vi "Process Menu Selection.vi"(8 "error in (no error)":errorcluster, 10 "Argument":string, 11 "Menu Ref":refnum<k9>) -> (0 "error out":errorcluster, 3 "State(s) to Enqueue":string)   [LabVIEW 2023, in "VI Properties Editor.lvlib"]
doc: "Processes a menu selection that occurred within the main window."
uses:
  VI Properties Editor.lvlib
  <vilib>/Utility/error.llb/Error Cluster From Error Code.vi
  <vilib>/ErrorRing/Error Ring.xnode
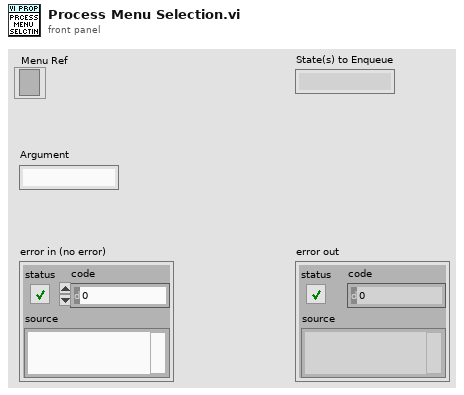
[diagram p1: front panel]
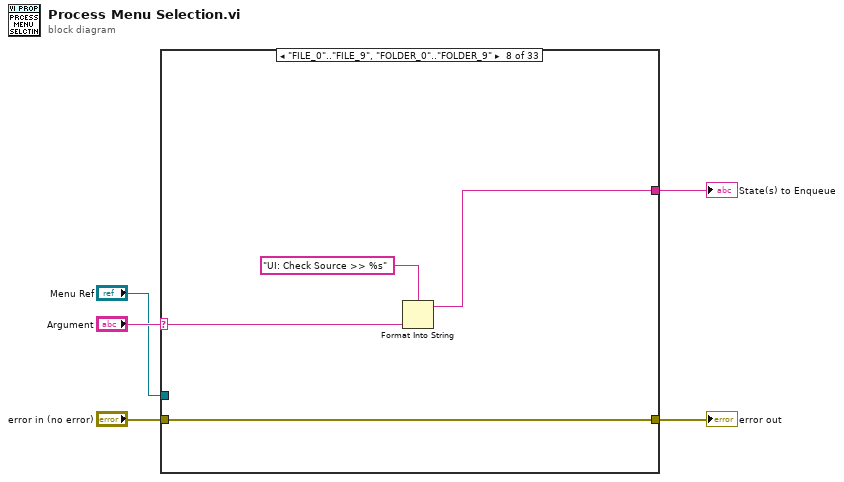
[diagram p0: block diagram]
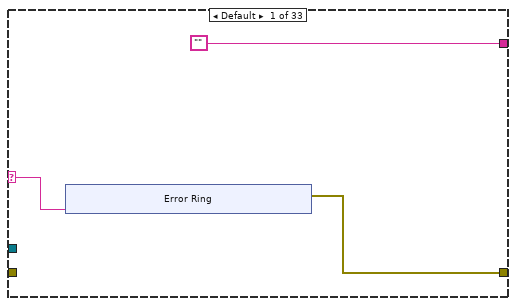
[diagram p2: hidden frame]
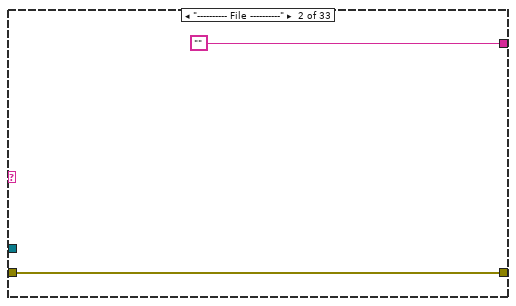
[diagram p3: hidden frame]
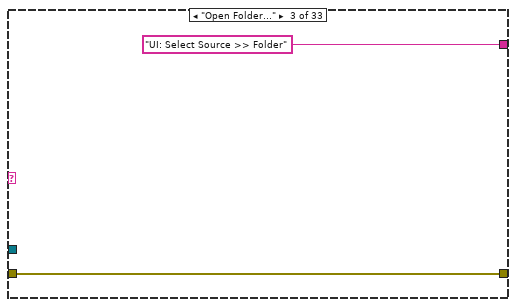
[diagram p4: hidden frame]
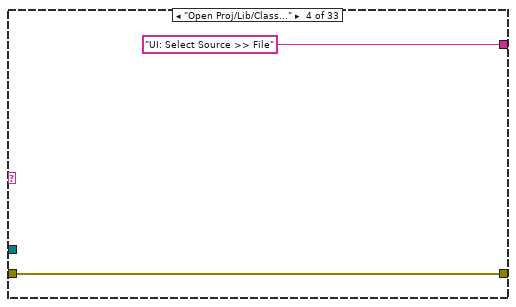
[diagram p5: hidden frame]
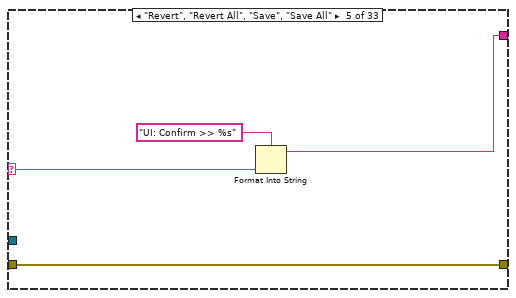
[diagram p6: hidden frame]
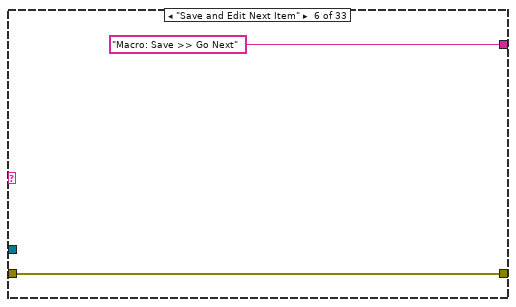
[diagram p7: hidden frame]
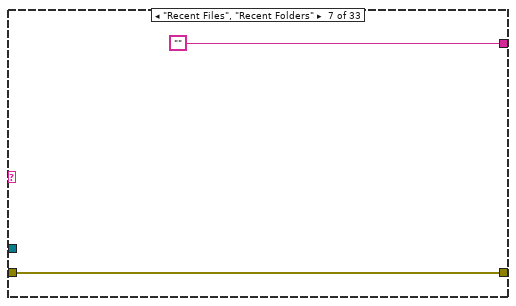
[diagram p8: hidden frame]
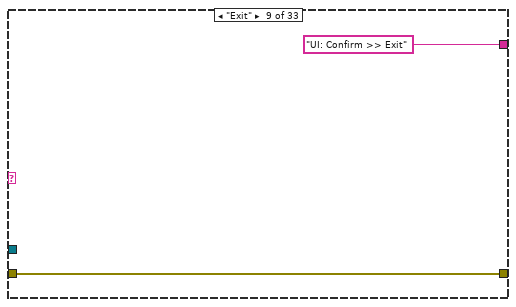
[diagram p9: hidden frame]
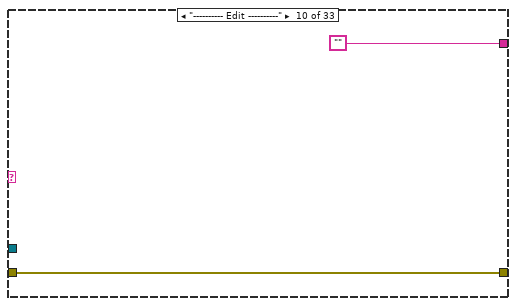
[diagram p10: hidden frame]
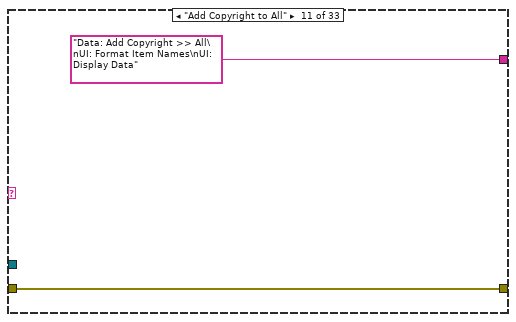
[diagram p11: hidden frame]
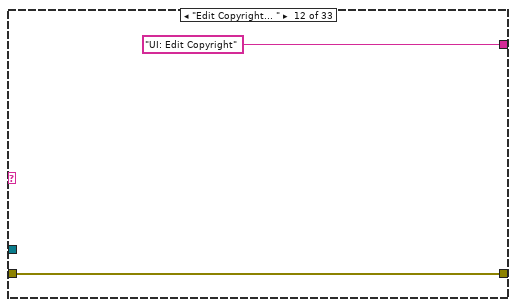
[diagram p12: hidden frame]
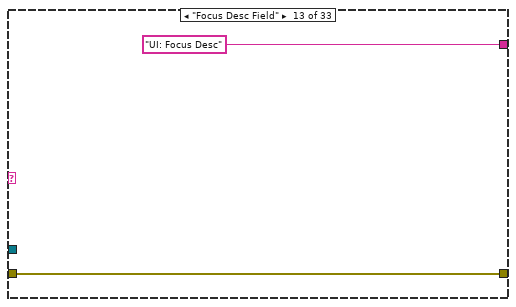
[diagram p13: hidden frame]
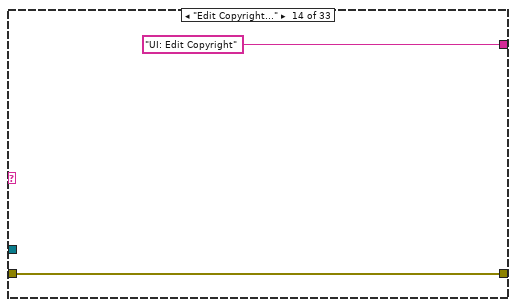
[diagram p14: hidden frame]
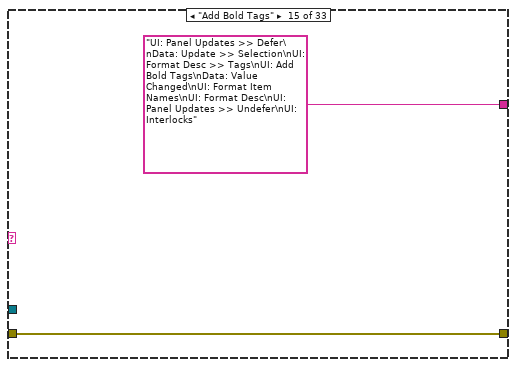
[diagram p15: hidden frame]
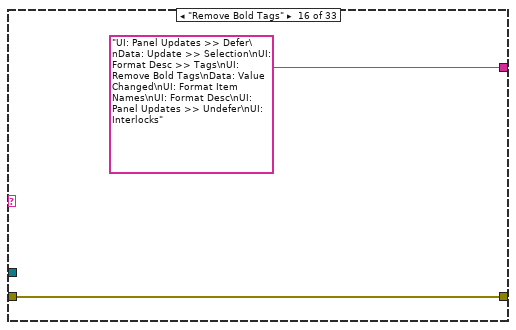
[diagram p16: hidden frame]
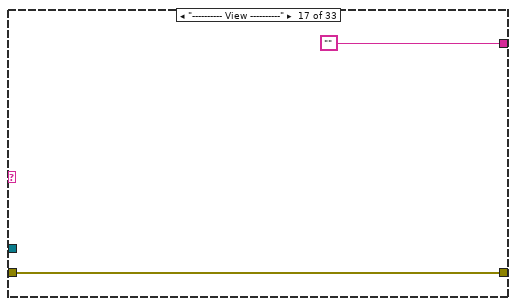
[diagram p17: hidden frame]
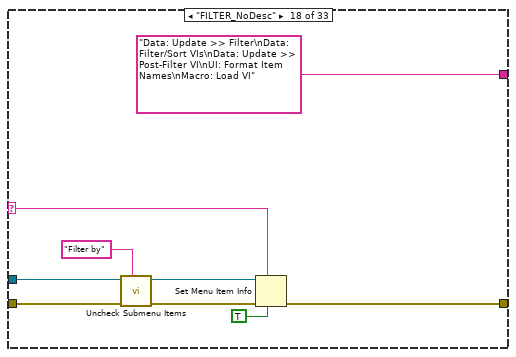
[diagram p18: hidden frame]
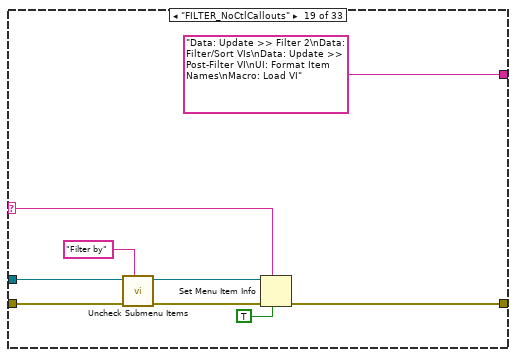
[diagram p19: hidden frame]
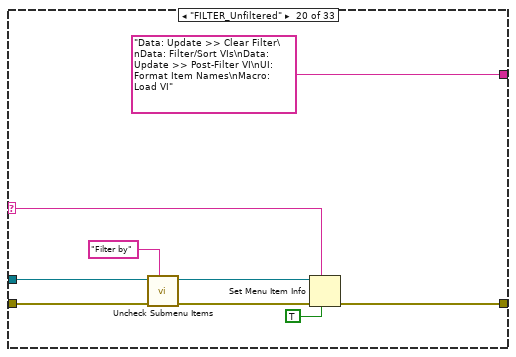
[diagram p20: hidden frame]
diagram:
  n1 = case shown="\"FILE_0\"..\"FILE_9\", \"FOLDER_0\"..\"FOLDER_9\"" "Argument" {
    selector: "Argument" -> [w6 _ _ _ w23 _ _ w30 _ _ _ _ _ _ _ _ _ w57 w66 w75 _ w82 _ w103 w113 w117 w132 w141 _ w152 w166 w175 _]
    tunnel: ["" "" "UI: Select Source >> Folder" "UI: Select Source >> File" w22 "Macro: Save >> Go Next" "" w31 "UI: Confirm >> Exit" "" "Data: Add Copyright >> All\nUI: Format Item Names\nUI: Display Data" "UI: Edit Copyright" "UI: Focus Desc" "UI: Edit Copyright" "UI: Panel Updates >> Defer\nData: Update >> Selection\nUI: Format Desc >> Tags\nUI: Add Bold Tags\nData: Value Changed\nUI: Format Item Names\nUI: Format Desc\nUI: Panel Updates >> Undefer\nUI: Interlocks" "UI: Panel Updates >> Defer\nData: Update >> Selection\nUI: Format Desc >> Tags\nUI: Remove Bold Tags\nData: Value Changed\nUI: Format Item Names\nUI: Format Desc\nUI: Panel Updates >> Undefer\nUI: Interlocks" "" "Data: Update >> Filter\nData: Filter/Sort VIs\nData: Update >> Post-Filter VI\nUI: Format Item Names\nMacro: Load VI" "Data: Update >> Filter 2\nData: Filter/Sort VIs\nData: Update >> Post-Filter VI\nUI: Format Item Names\nMacro: Load VI" "Data: Update >> Clear Filter\nData: Filter/Sort VIs\nData: Update >> Post-Filter VI\nUI: Format Item Names\nMacro: Load VI" "UI: Add Custom Filter" "Data: Update >> Filter Config\nData: Write Config\nUI: Initialize Menu\nData: Filter/Sort VIs\nData: Update >> Post-Filter VI\nUI: Format Item Names\nMacro: Load VI" "" w105 "Data: Update >> Filter Data Source\nData: Filter/Sort VIs\nData: Update >> Post-Filter VI\nUI: Format Item Names\nMacro: Load VI" w116 "Data: Update >> Unsort\nData: Filter/Sort VIs\nData: Update >> Post-Filter VI\nUI: Format Item Names\nMacro: Load VI" "Data: Update >> Sort Order\nData: Filter/Sort VIs\nData: Update >> Post-Filter VI\nUI: Format Item Names\nMacro: Load VI" "" "Data: Update >> Abbr Names?\nUI: Format Item Names\nData: Write Config" w157 "Data: Update >> ShowCPCtlsOnly?\nData: Write Config\nData: Update >> All Ctls\nUI: Display Data" "UI: Edit Options"] -> w5
    tunnel: "Menu Ref" -> [_ _ _ _ _ _ _ _ _ _ _ _ _ _ _ _ _ w54 w63 w73 _ w88 _ w94 w114 w121 w133 w142 _ w153 w167 w176 _]
    tunnel: "error in (no error)" -> [_ w16 w18 w20 w25 w26 w28 w33 w35 w37 w38 w40 w42 w44 w46 w48 w51 w58 w67 w76 w79 w90 w92 w97 w108 w122 w131 w138 w145 w147 w162 w171 w177]
    tunnel: [w7 w16 w18 w20 w25 w26 w28 w33 w35 w37 w38 w40 w42 w44 w46 w48 w51 w56 w65 w70 w79 w85 w92 w96 w107 w125 w130 w137 w145 w146 w161 w170 w177] -> w4
    frame Default {
      n2 = xnode "Error Ring"("parameter 0"=w6) -> ("error out"=w7:errorcluster)
    }
    frame "---------- File ----------" {
    }
    frame "Open Folder..." {
    }
    frame "Open Proj/Lib/Class..." {
    }
    frame "Revert", "Revert All", "Save", "Save All" {
      n3 = Format Into String(format string="UI: Confirm >> %s", w23) -> (resulting string=w22:string)  [unwired: 2 in, 1 out]
    }
    frame "Save and Edit Next Item" {
    }
    frame "Recent Files", "Recent Folders" {
    }
    frame "FILE_0".."FILE_9", "FOLDER_0".."FOLDER_9" {
      n4 = Format Into String(format string="UI: Check Source >> %s", w30) -> (resulting string=w31:string)  [unwired: 2 in, 1 out]
    }
    frame "Exit" {
    }
    frame "---------- Edit ----------" {
    }
    frame "Add Copyright to All" {
    }
    frame "Edit Copyright... " {
    }
    frame "Focus Desc Field" {
    }
    frame "Edit Copyright..." {
    }
    frame "Add Bold Tags" {
    }
    frame "Remove Bold Tags" {
    }
    frame "---------- View ----------" {
    }
    frame "FILTER_NoDesc" {
      n5 = call "Uncheck Submenu Items.vi"("Item Tag"="Filter by", "error in (no error)"=w58, "Menu Ref"=w54) -> ("error out"=w55:errorcluster, "Menu Ref out"=w53:refnum<k9>)  [unwired: 7 in]
      n6 = Set Menu Item Info(6:TRUE ("checked"), 7:w57, 8:w55, 11:w53) -> (0:w56:errorcluster)  [unwired: 3 in, 1 out]
    }
    frame "FILTER_NoCtlCallouts" {
      n7 = call "Uncheck Submenu Items.vi"("Item Tag"="Filter by", "error in (no error)"=w67, "Menu Ref"=w63) -> ("error out"=w64:errorcluster, "Menu Ref out"=w62:refnum<k9>)  [unwired: 7 in]
      n8 = Set Menu Item Info(6:TRUE ("checked"), 7:w66, 8:w64, 11:w62) -> (0:w65:errorcluster)  [unwired: 3 in, 1 out]
    }
    frame "FILTER_Unfiltered" {
      n9 = call "Uncheck Submenu Items.vi"("Item Tag"="Filter by", "error in (no error)"=w76, "Menu Ref"=w73) -> ("error out"=w74:errorcluster, "Menu Ref out"=w72:refnum<k9>)  [unwired: 7 in]
      n10 = Set Menu Item Info(6:TRUE ("checked"), 7:w75, 8:w74, 11:w72) -> (0:w70:errorcluster)  [unwired: 3 in, 1 out]
    }
    frame "FILTER_Custom" {
    }
    frame "FILTER_Custom_Do" {
      n11 = call "Uncheck Submenu Items.vi"("Item Tag"="Filter by", "error in (no error)"=w90, "Menu Ref"=w88) -> ("error out"=w89:errorcluster, "Menu Ref out"=w87:refnum<k9>)  [unwired: 7 in]
      n12 = Search/Split String(string=w82, search string/char (-)="_Do") -> (substring before match=w81:string)  [unwired: 1 in, 2 out]
      n13 = Set Menu Item Info(6:TRUE ("checked"), 7:w81, 8:w89, 11:w87) -> (0:w85:errorcluster)  [unwired: 3 in, 1 out]
    }
    frame "Recent Filters" {
    }
    frame "FILTER_0".."FILTER_9" {
      n14 = Search/Split String(string=w103, search string/char (-)="_") -> (substring before match=w104:string)  [unwired: 1 in, 2 out]
      n15 = call "Uncheck Submenu Items.vi"("Item Tag"="Filter by", "error in (no error)"=w97, "Menu Ref"=w94) -> ("error out"=w101:errorcluster, "Menu Ref out"=w100:refnum<k9>)  [unwired: 7 in]
      n16 = Format Into String(format string="Data: Update >> %s\nData: Update >> %s Config\nData: Write Config\nData: Filter/Sort VIs\nData: Update >> Post-Filter VI\nUI: Format Item Names\nMacro: Load VI", w103, w104) -> (resulting string=w105:string)  [unwired: 2 in, 1 out]
      n17 = Set Menu Item Info(6:TRUE ("checked"), 7:"FILTER_Custom" ("item tag"), 8:w101, 11:w100) -> (0:w96:errorcluster)  [unwired: 3 in, 1 out]
    }
    frame "FILTER_DataSource" {
      n18 = Get Menu Item Info(7:w113, 8:w108, 11:w114) -> (0:w112:errorcluster, 3:w111:refnum<k9>, 4:w110:bool)  [unwired: 4 out]
      n19 = Not(x=w110) -> (.not. x?=w109:bool)
      n20 = Set Menu Item Info(6:w109, 7:w113, 8:w112, 11:w111) -> (0:w107:errorcluster)  [unwired: 3 in, 1 out]
    }
    frame "SORT_0".."SORT_99" {
      n21 = call "Uncheck Submenu Items.vi"("Item Tag"="Sort by" ("item tag"), "error in (no error)"=w122, "Menu Ref"=w121) -> ("error out"=w119:errorcluster, "Menu Ref out"=w120:refnum<k9>)  [unwired: 7 in]
      n22 = Set Menu Item Info(6:TRUE ("checked"), 7:w117, 8:w119, 11:w120) -> (0:w125:errorcluster)  [unwired: 3 in, 1 out]
      n23 = Format Into String(format string="Data: Update >> %s\nData: Filter/Sort VIs\nData: Update >> Post-Filter VI\nUI: Format Item Names\nMacro: Load VI", w117) -> (resulting string=w116:string)  [unwired: 2 in, 1 out]
    }
    frame "SORT_Unsorted" {
      n24 = call "Uncheck Submenu Items.vi"("Item Tag"="Sort by" ("item tag"), "error in (no error)"=w131, "Menu Ref"=w133) -> ("error out"=w126:errorcluster, "Menu Ref out"=w127:refnum<k9>)  [unwired: 7 in]
      n25 = Set Menu Item Info(6:TRUE ("checked"), 7:w132, 8:w126, 11:w127) -> (0:w130:errorcluster)  [unwired: 3 in, 1 out]
    }
    frame "SORT_Order" {
      n26 = Get Menu Item Info(7:w141, 8:w138, 11:w142) -> (0:w140:errorcluster, 3:w139:refnum<k9>, 4:w136:bool)  [unwired: 4 out]
      n27 = Not(x=w136) -> (.not. x?=w135:bool)
      n28 = Set Menu Item Info(6:w135, 7:w141, 8:w140, 11:w139) -> (0:w137:errorcluster)  [unwired: 3 in, 1 out]
    }
    frame "---------- Options ----------" {
    }
    frame "Abbr if Class in Lib" {
      n29 = Get Menu Item Info(7:w152, 8:w147, 11:w153) -> (0:w151:errorcluster, 3:w150:refnum<k9>, 4:w149:bool)  [unwired: 4 out]
      n30 = Not(x=w149) -> (.not. x?=w148:bool)
      n31 = Set Menu Item Info(6:w148, 7:w152, 8:w151, 11:w150) -> (0:w146:errorcluster)  [unwired: 3 in, 1 out]
    }
    frame "Format Bold Text" {
      n32 = Get Menu Item Info(7:w166, 8:w162, 11:w167) -> (0:w165:errorcluster, 3:w164:refnum<k9>, 4:w163:bool)  [unwired: 4 out]
      n33 = Not(x=w163) -> (.not. x?=w160:bool)
      n34 = Set Menu Item Info(6:w160, 7:w166, 8:w165, 11:w164) -> (0:w161:errorcluster)  [unwired: 3 in, 1 out]
      n35 = Select(t="UI: Format Desc", s=w160, f="UI: Format Desc >> Tags") -> (s? t:f=w155:string)
      n36 = Format Into String(format string="Data: Update >> Format Bold?\nData: Write Config\nUI: Display Data\n%s", w155) -> (resulting string=w157:string)  [unwired: 2 in, 1 out]
    }
    frame "Only Show ConPane Ctls" {
      n37 = Get Menu Item Info(7:w175, 8:w171, 11:w176) -> (0:w174:errorcluster, 3:w173:refnum<k9>, 4:w172:bool)  [unwired: 4 out]
      n38 = Not(x=w172) -> (.not. x?=w169:bool)
      n39 = Set Menu Item Info(6:w169, 7:w175, 8:w174, 11:w173) -> (0:w170:errorcluster)  [unwired: 3 in, 1 out]
    }
    frame "All Options..." {
    }
  }
  "error out" <- w4
  "State(s) to Enqueue" <- w5
